vi "hit_pos.vi"(2 "radius":dbl=12.0 format="%#_13g", 3 "TARGET Circle Descriptor":T1, 4 "GOALpos":cluster{"X":sgl, "Y":sgl}={"X"=100.0, "Y"=100.0}) -> (0 "endX":dbl format="%#_13g", 1 "endY":dbl format="%#_13g")   [LabVIEW 2018]
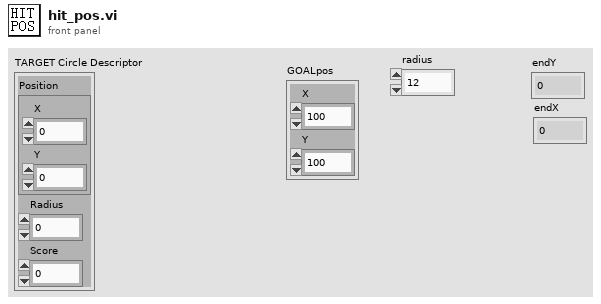
[diagram p1: front panel]
types:
  T1 = cluster{"Position":cluster{"X":sgl, "Y":sgl}, "Radius":dbl, "Score":dbl}
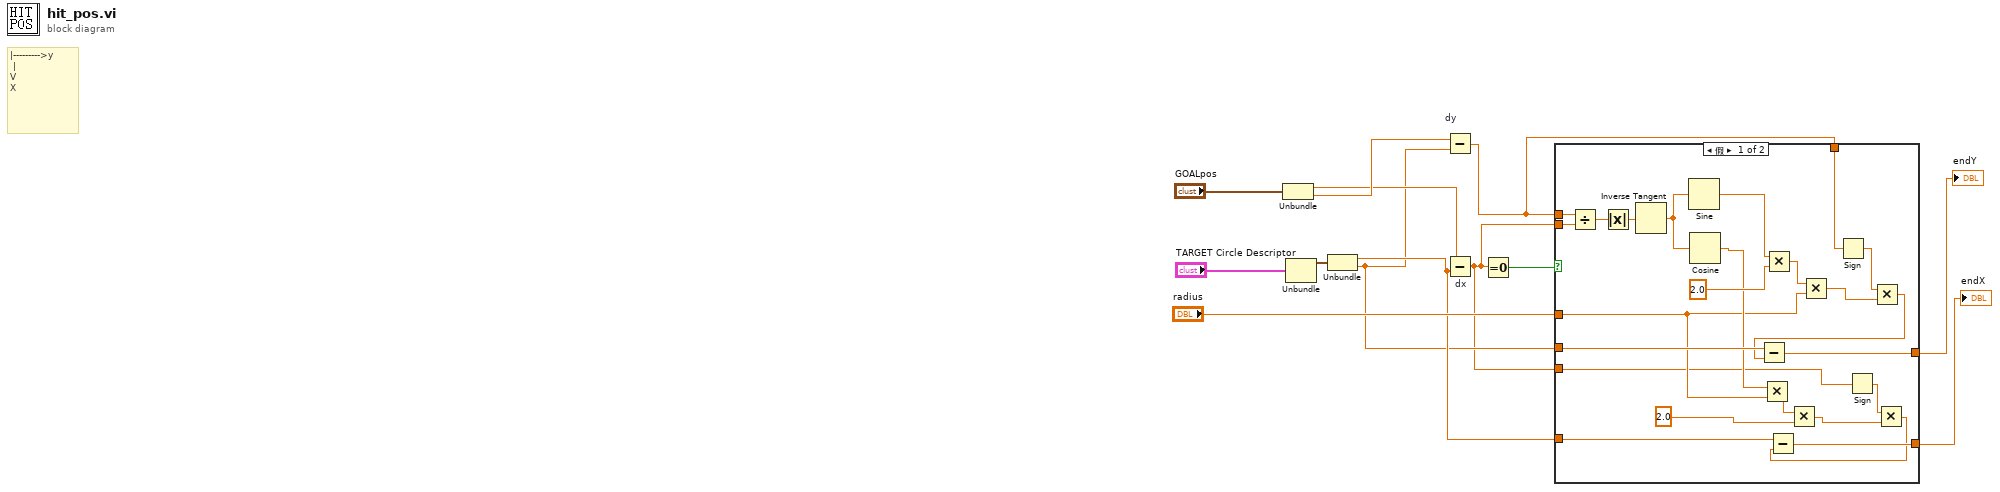
[diagram p0: block diagram]
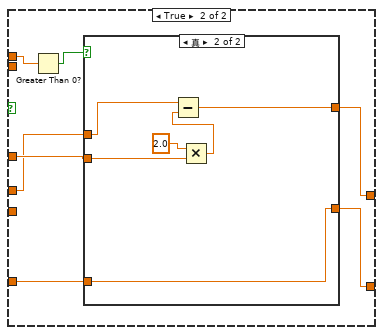
[diagram p2: hidden frame]
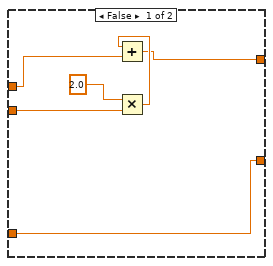
[diagram p3: hidden frame]
diagram:
  # "|--------->y\n |\nV\nX"
  n1 = Unbundle("GOALpos") -> ("X"=w12:sgl, "Y"=w13:sgl)
  n2 = Unbundle("TARGET Circle Descriptor") -> ("Position"=w1:cluster{"X":sgl, "Y":sgl})  [unwired: 2 out]
  n3 = Unbundle(w1) -> ("X"=w9:sgl, "Y"=w8:sgl)
  n4 = Subtract "dy"(x=w13, y=w8) -> (x-y=w7:sgl)
  n5 = Subtract "dx"(x=w12, y=w9) -> (x-y=w4:sgl)
  n6 = Equal To 0?(x=w4) -> (x = 0?=w11:bool)
  n7 = case shown="假" w11 {
    tunnel: [w33 w41] -> w6
    tunnel: [w31 w39] -> w5
    tunnel: w7 -> [w37 w44]
    tunnel: w4 -> [w36 _]
    tunnel: w8 -> [w34 w38]
    tunnel: "radius" -> [w26 w42]
    tunnel: w9 -> [w32 w40]
    tunnel: w7 -> [w20 _]
    tunnel: w4 -> [w14 _]
    frame False {
      n8 = Divide(x=w37, y=w36) -> (x/y=w16:sgl)
      n9 = Absolute Value(x=w16) -> (abs(x)=w15:sgl)
      n10 = Inverse Tangent(1:w15) -> (0:w35:sgl)
      n11 = Sine(x=w35) -> (sin(x)=w30:sgl)
      n12 = Cosine(x=w35) -> (cos(x)=w27:sgl)
      n13 = Multiply(x=w27, y=w26) -> (x*y=w25:dbl)
      n14 = Multiply(x=w30, y=2.0) -> (x*y=w28:dbl)
      n15 = Multiply(x=w25, y=2.0) -> (x*y=w18:dbl)
      n16 = Multiply(x=w28, y=w26) -> (x*y=w22:dbl)
      n17 = Sign(1:w20) -> (0:w23:sgl)
      n18 = Sign(1:w14) -> (0:w19:sgl)
      n19 = Multiply(x=w23, y=w22) -> (x*y=w21:dbl)
      n20 = Subtract(x=w34, y=w21) -> (x-y=w33:dbl)
      n21 = Multiply(x=w19, y=w18) -> (x*y=w17:dbl)
      n22 = Subtract(x=w32, y=w17) -> (x-y=w31:dbl)
    }
    frame True {
      n23 = Greater Than 0?(x=w44) -> (x > 0?=w43:bool)
      n24 = case shown="真" w43 {
        tunnel: w42 -> [w46 w52]
        tunnel: w38 -> [w49 w55]
        tunnel: [w47 w53] -> w41
        tunnel: w40 -> [w45 w51]
        tunnel: [w45 w51] -> w39
        frame False {
          n25 = Multiply(x=2.0, y=w46) -> (x*y=w48:dbl)
          n26 = Add(x=w48, y=w49) -> (x+y=w47:dbl)
        }
        frame True {
          n27 = Multiply(x=2.0, y=w52) -> (x*y=w54:dbl)
          n28 = Subtract(x=w55, y=w54) -> (x-y=w53:dbl)
        }
      }
    }
  }
  "endY" <- w6
  "endX" <- w5
